vi "GCMPlugin_IsSupportingItem.vi"(8 "error in (no error)":errorcluster, 9 "VI Reference":refnum<vi>, 10 "ProjectItem Refnum":refnum<vi>, 11 "_LVCMPlugin in":refnum<class "GCMPlugin.lvclass">) -> (0 "error out":errorcluster, 2 "IsSupportingItem":bool, 3 "_LVCMPlugin out":refnum<class "GCMPlugin.lvclass">)   [LabVIEW 2014, in "GCMPlugin.lvclass"]
uses:
  GCMPlugin/GCMPlugin.lvclass
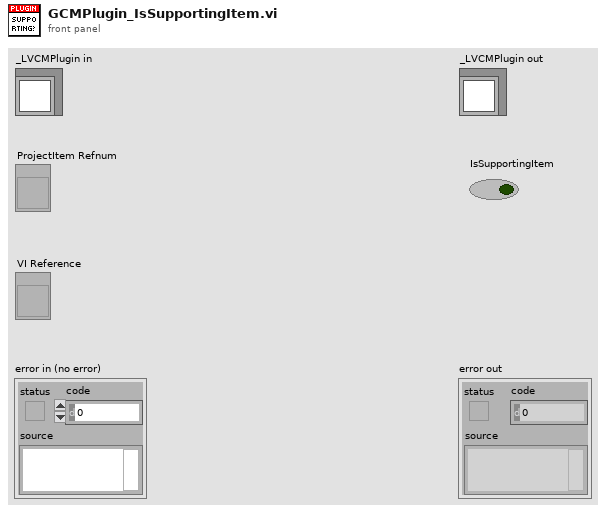
[diagram p1: front panel]
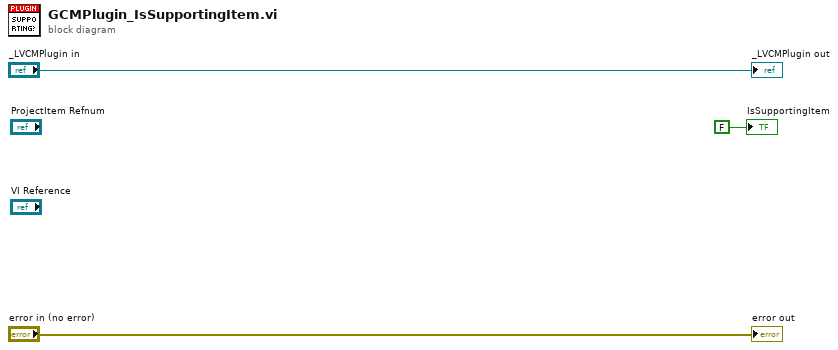
[diagram p0: block diagram]
diagram:
  "error out" <- "error in (no error)"
  "_LVCMPlugin out" <- "_LVCMPlugin in"
  "IsSupportingItem" <- FALSE ("IsSupportingItem")
